vi "Register Test.vi"(6 "Call Chain":string[](array[string]), 7 "Caller ID":string, 8 "error in (no error)":errorcluster, 9 "Test ID":string, 10 "Name":string, 11 "Test Manager in":refnum<class "Basic Test Manager.lvclass">) -> (0 "error out":errorcluster, 3 "Test Manager out":refnum<class "Basic Test Manager.lvclass">)   [LabVIEW 2013, in "Caraya.lvlib" / "Basic Test Manager.lvclass"]
uses:
  Basic Test Manager.lvclass
  Test Result/Test Event Data.ctl
  Test Result/Test Registration Data.ctl
  Basic Test Manager.lvclass/Basic Test Manager.ctl
  Test Result/Test Result.lvclass
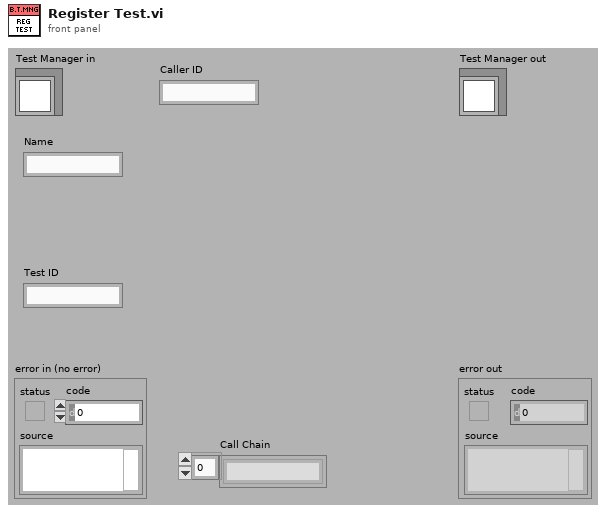
[diagram p1: front panel]
types:
  T1 = typedef "Caraya.lvlib/Test Result.lvclass/Test Registration Data.ctl" = cluster{"Name":string, "Call Chain":string[], "Time Stamp":timestamp, "Test ID":string, "Caller ID":string}
  T2 = typedef "Caraya.lvlib/Test Result.lvclass/Test Event Data.ctl" = cluster{"Label":string, "Argument":variant}
  T3 = typedef "Caraya.lvlib/Test Result.lvclass/Test Event.ctl" = refnum<user-event>
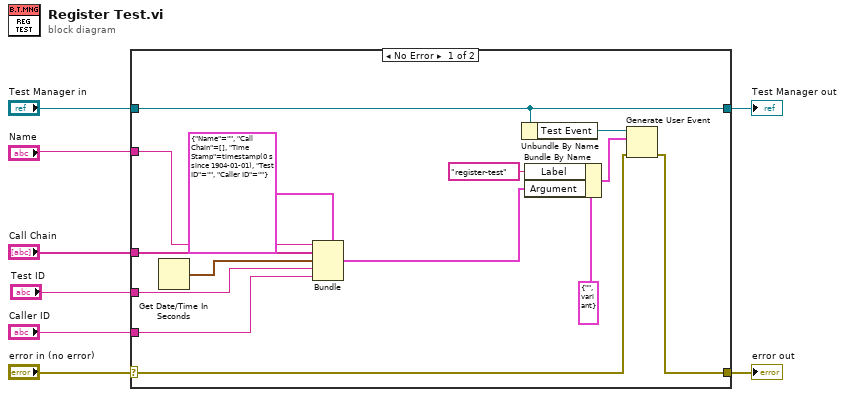
[diagram p0: block diagram]
diagram:
  n1 = case shown="No Error" "error in (no error)" {
    selector: "error in (no error)" -> [w18 w24]
    tunnel: [w17 w24] -> w7
    tunnel: [w20 w23] -> w5
    tunnel: "Test Manager in" -> [w20 w23]
    tunnel: "Name" -> [w22 _]
    tunnel: "Call Chain" -> [w21 _]
    tunnel: "Test ID" -> [w10 _]
    tunnel: "Caller ID" -> [w9 _]
    frame No Error {
      n2 = Get Date/Time In Seconds() -> (seconds since 1Jan1904=w11:timestamp)
      n3 = Bundle(cluster=T1 {"Name"="", "Call Chain"=[], "Time Stamp"=timestamp(0 s since 1904-01-01), "Test ID"="", "Caller ID"=""} ("Test Registration"), "Name"=w22, "Call Chain"=w21, "Time Stamp"=w11, "Test ID"=w10, "Caller ID"=w9) -> (w13:T1)
      n4 = Unbundle By Name(w20) -> ("Test Event"=w19:T3)
      n5 = Bundle By Name(cluster=T2 {"Label"="", "Argument"=variant} ("event data"), "Label"="register-test" ("Message"), "Argument"=w13) -> (w15:T2)
      n6 = Generate User Event(user event=w19, event data cluster=w15, error in=w18) -> (error out=w17:errorcluster)  [unwired: 1 in, 1 out]
    }
    frame Error {
    }
  }
  "error out" <- w7
  "Test Manager out" <- w5
